vi "OEE_SCREEN_1_recolor_cycle_time_actual.vi"(1 "cycle_time_actual_field_reference":refnum<vi>, 2 "cycle_time_actual":string, 3 "cycle_time_target":string) -> ()   [LabVIEW 2019]
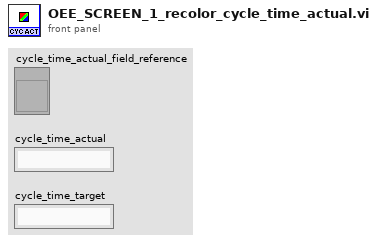
[diagram p1: front panel]
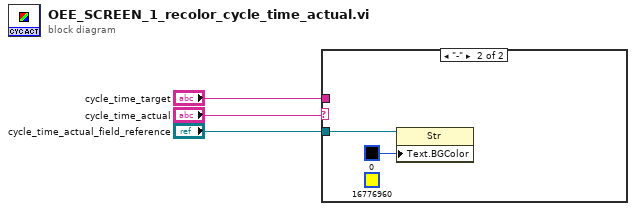
[diagram p0: block diagram]
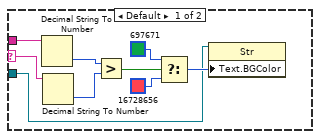
[diagram p2: hidden frame]
diagram:
  n1 = case shown="\"-\"" "cycle_time_actual" {
    selector: "cycle_time_actual" -> [w11 _]
    tunnel: "cycle_time_actual_field_reference" -> [w6 w14]
    tunnel: "cycle_time_target" -> [w12 _]
    frame Default {
      n2 = Decimal String To Number(string=w12) -> (number=w9:i32)  [unwired: 2 in, 1 out]
      n3 = Decimal String To Number(string=w11) -> (number=w8:i32)  [unwired: 2 in, 1 out]
      n4 = Greater?(x=w9, y=w8) -> (0:w10:bool)
      n5 = Select(t=u32 697671, s=w10, f=u32 16728656) -> (s? t:f=w7:u32)
      n6 = property class="Str"(reference=w6, "Text.BGColor"=w7) -> ()  [unwired: 1 in, 2 out]
    }
    frame "-" {
      (unwired) u32 16776960
      n7 = property class="Str"(reference=w14, "Text.BGColor"=u32 0) -> ()  [unwired: 1 in, 2 out]
    }
  }
